vi "replymessage.vi"(2 "error in (no error)":errorcluster, 3 "retcode":u16(ring) items=["0"=0, "1"=1, "100"=100, "101"=101, "102"=102, "200"=200, "201"=202, "300"=300, "301"=301, "302"=302, "303"=303, "304"=304, "305"=305, "306"=306, "307"=307, "308"=308, "309"=309, "400"=400, "500"=500, "501"=501, "502"=502, "999"=999], 4 "input json string":string="{\"values_raw\": 1}") -> (0 "error out":errorcluster, 1 "body":string)   [LabVIEW 2016]
doc: "Format the message to follow dripline standard"
panel:
  in  "return_msg":string
  out "sender_info":T1
  out "timestamp":string
  in  "package":string="dripline"
  in  "commit":string="xxxxx"
  in  "version":string="v0.0.0"
  in  "service_name":string="dripline"
  out "exe":string
  out "username":string
  out "hostname":string
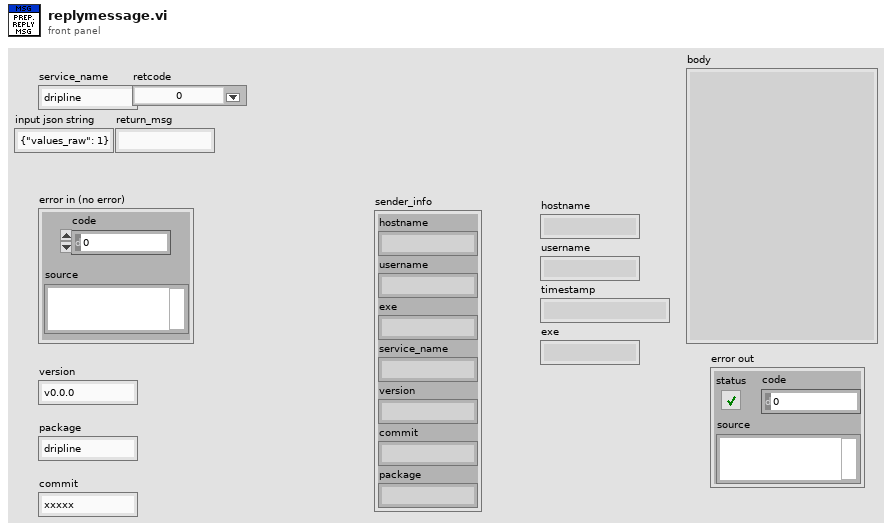
[diagram p1: front panel]
types:
  T1 = cluster{"hostname":string, "username":string, "exe":string, "service_name":string, "version":string, "commit":string, "package":string}
  T2 = cluster{"timestamp":string, "retcode":u16, "return_msg":string, "sender_info":cluster{"hostname":string, "username":string, "exe":string, "service_name":string, "version":string, "commit":string, "package":string}, "msgtype":i32}
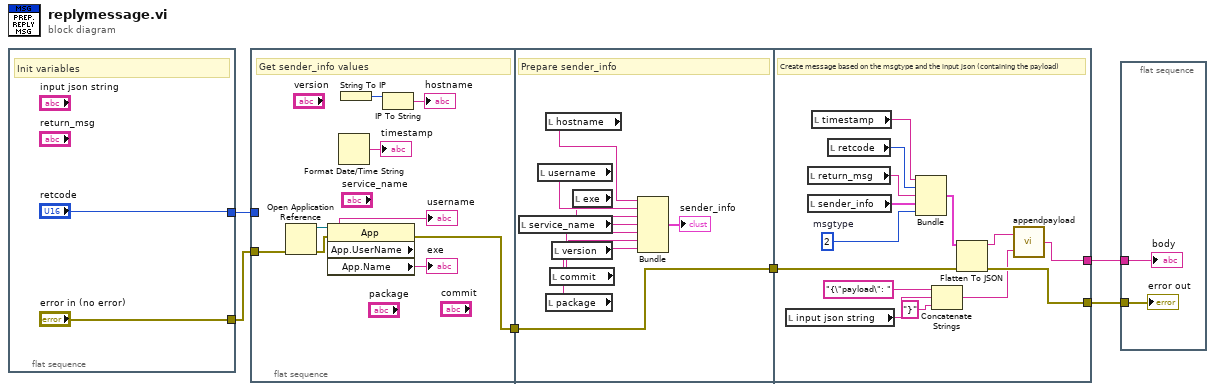
[diagram p0: block diagram]
diagram:
  n1 = flat-sequence {
    tunnel: ["error in (no error)"] -> w3
    tunnel: ["retcode"] -> w4
    frame #0 {
      # "Init variables"
    }
  }
  n2 = flat-sequence {
    tunnel: w4 -> [_]
    tunnel: w3 -> [w11]
    tunnel: [w9] -> w1
    tunnel: [w18] -> w2
    tunnel: w1 -> [w18]
    tunnel: [w39] -> w6
    tunnel: [w35] -> w5
    tunnel: w2 -> [w27]
    frame #0 {
      # "Get sender_info values"
      n3 = Open Application Reference(8:w11) -> (0:w10:errorcluster, 3:w14:refnum<vi>)  [unwired: 3 in]
      n4 = property class="App"(reference=w14, error in=w10) -> (error out=w9:errorcluster, "App.UserName"=→"username":string, "App.Name"=→"exe":string)  [unwired: 1 out]
      n5 = Format Date/Time String() -> (date/time string=→"timestamp":string)  [unwired: 3 in]
      n6 = String To IP() -> (0:w15:u32)  [unwired: 1 in]
      n7 = IP To String(2:w15) -> (0:→"hostname":string)  [unwired: 1 in]
    }
    frame #1 {
      # "Prepare sender_info"
      n8 = local read "service_name"() -> (w23:string)
      n9 = local read "username"() -> (w26:string)
      n10 = local read "hostname"() -> (w25:string)
      n11 = local read "package"() -> (w20:string)
      n12 = local read "commit"() -> (w21:string)
      n13 = local read "version"() -> (w22:string)
      n14 = local read "exe"() -> (w24:string)
      n15 = Bundle("hostname"=w25, "username"=w26, "exe"=w24, "service_name"=w23, "version"=w22, "commit"=w21, "package"=w20) -> (→"sender_info":T1)  [unwired: 1 in]
    }
    frame #2 {
      w28 = 2  # msgtype
      # "Create message based on the msgtype and the input json (containing the payload)"
      n16 = local read "input json string"() -> (w30:string)
      n17 = local read "return_msg"() -> (w34:string)
      n18 = local read "sender_info"() -> (w38:T1)
      n19 = local read "timestamp"() -> (w40:string)
      n20 = local read "retcode"() -> (w37:u16)
      n21 = Bundle("timestamp"=w40, "retcode"=w37, "return_msg"=w34, "sender_info"=w38, "msgtype"=w28) -> (w29:T2)  [unwired: 1 in]
      n22 = Concatenate Strings("{\"payload\": " ("string"), w30, "}" ("string")) -> (w31:string)
      n23 = Flatten To JSON(anything=w29, error in (no error)=w27) -> (JSON string=w36:string, 11:w39:errorcluster)  [unwired: 1 in]
      n24 = call "appendpayload.vi"("jsontoappend"=w31, "basejson"=w36) -> ("concatenated json string"=w35:string)
    }
  }
  n25 = flat-sequence {
    tunnel: w6 -> [w42]
    tunnel: w5 -> [w41]
    frame #0 {
      "error out" <- w42
      "body" <- w41
    }
  }
